vi "buildWorkerStartNew.vi"(8 "error in (no error)":errorcluster, 11 "BuildServer in":refnum<class "BuildServer.lvclass">) -> (0 "error out":errorcluster, 3 "BuildServer out":refnum<class "BuildServer.lvclass">)   [LabVIEW 2017, in "BuildServer.lvlib" / "BuildServer.lvclass"]
uses:
  BuildServer.lvclass
  BuildServer.lvclass/BuildServer.ctl
  BuildWorker/Classes/BuildWorker/BuildWorker.lvclass
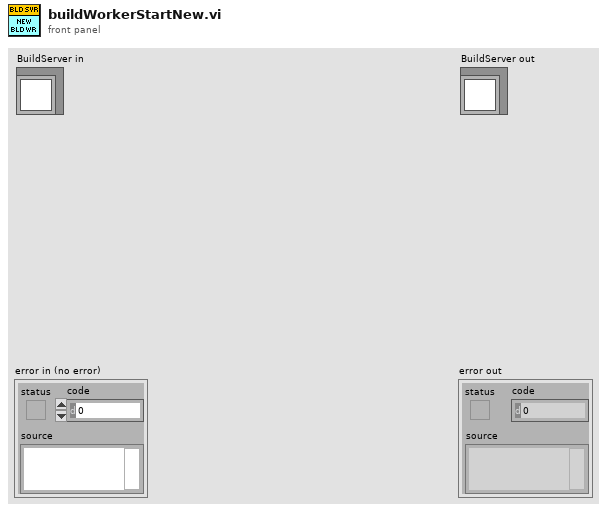
[diagram p1: front panel]
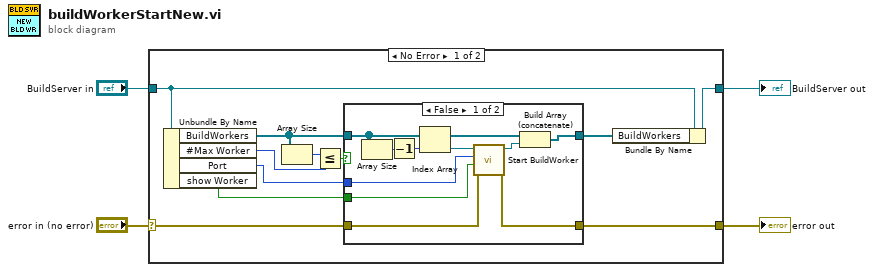
[diagram p0: block diagram]
diagram:
  n1 = case shown="No Error" "error in (no error)" {
    selector: "error in (no error)" -> [w15 w29]
    tunnel: [w14 w29] -> w3
    tunnel: [w11 w28] -> w1
    tunnel: "BuildServer in" -> [w13 w28]
    frame No Error {
      n2 = Unbundle By Name(w13) -> ("BuildWorkers"=w12:refnum<class "BuildWorker.lvclass">[], "#Max Worker"=w8:i32, "Port"=w6:u16, "show Worker"=w5:bool)
      n3 = Array Size(array=w12) -> (size(s)=w9:i32)
      n4 = Less Or Equal?(x=w9, y=w8) -> (x <= y?=w7:bool)
      n5 = case shown="False" w7 {
        tunnel: w15 -> [w19 w26]
        tunnel: [w21 w26] -> w14
        tunnel: w12 -> [w24 w27]
        tunnel: [w25 w27] -> w10
        tunnel: w6 -> [w17 _]
        tunnel: w5 -> [w16 _]
        frame False {
          n6 = Array Size(array=w24) -> (size(s)=w23:i32)
          n7 = Decrement(x=w23) -> (x-1=w22:i32)
          n8 = Index Array(array=w24, index=w22) -> (element=w18:refnum<class "BuildWorker.lvclass">)
          n9 = call-dynamic "Start BuildWorker.vi"("error in (no error)"=w19, "Show"=w16, "Port"=w17, "BuildWorker in"=w18) -> ("error out"=w21:errorcluster, "BuildWorker out"=w20:refnum<class "BuildWorker.lvclass">)  [unwired: 6 in]
          n10 = Build Array (concatenate)(w24, w20) -> (w25:refnum<class "BuildWorker.lvclass">[])
        }
        frame True {
        }
      }
      n11 = Bundle By Name(cluster=w13, "BuildWorkers"=w10) -> (w11:refnum<class "BuildServer.lvclass">)
    }
    frame Error {
    }
  }
  "error out" <- w3
  "BuildServer out" <- w1
